vi "CRYWindow WAIT FRAME.vi"(7 "sAction":string, 10 "vi reference":refnum<vi>) -> (1 "sData_Out":string)   [LabVIEW 2013]
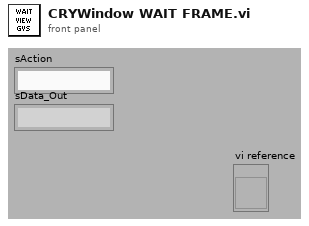
[diagram p1: front panel]
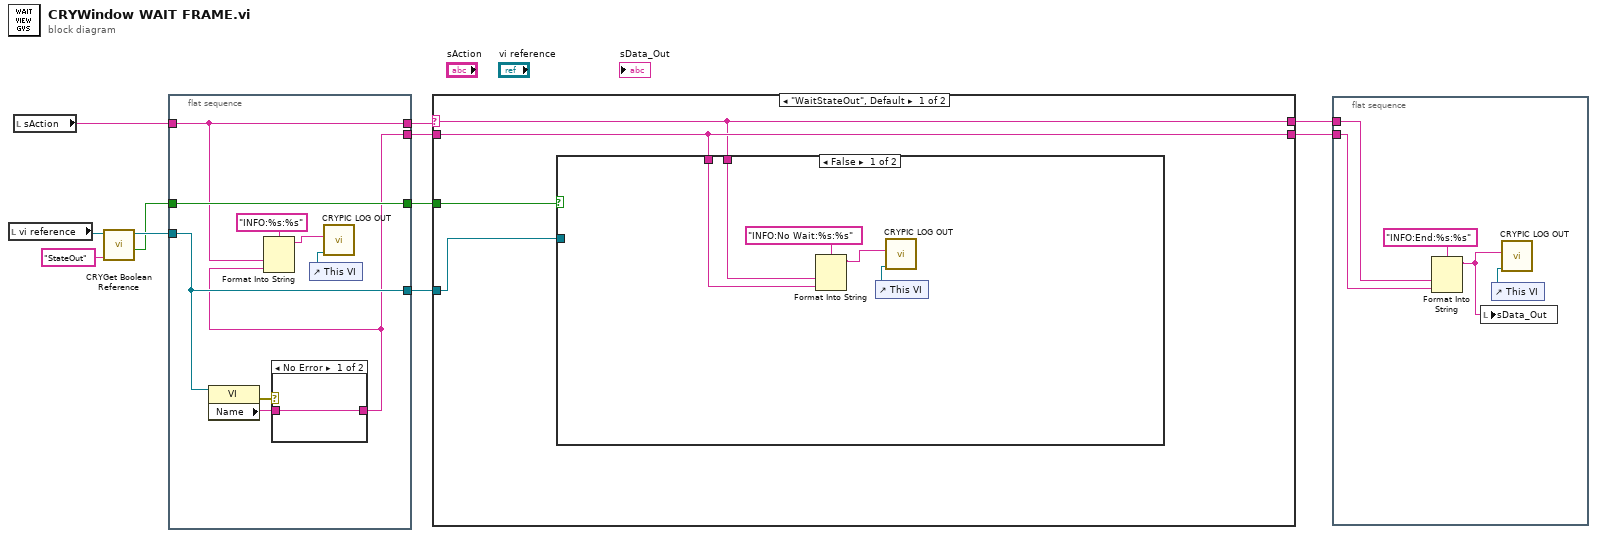
[diagram p0: block diagram]
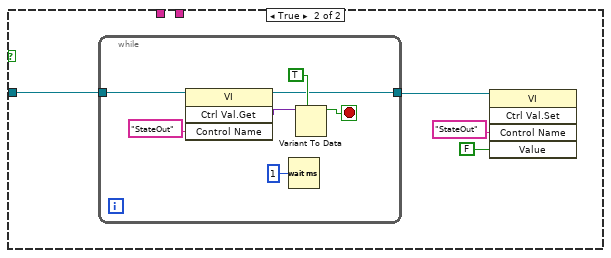
[diagram p2: hidden frame]
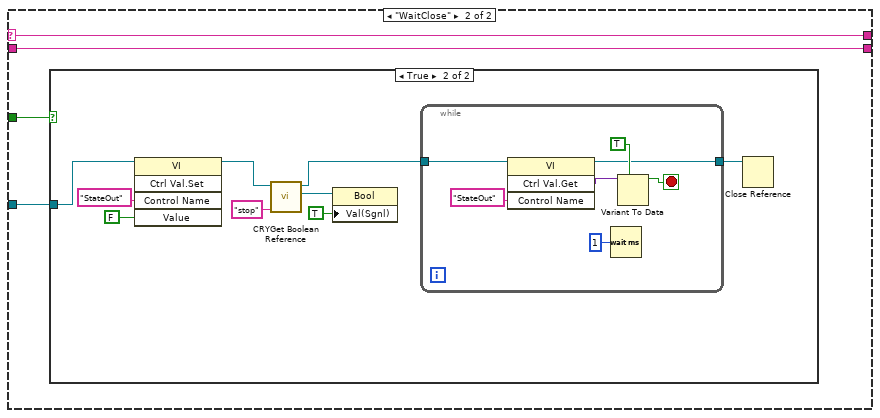
[diagram p3: hidden frame]
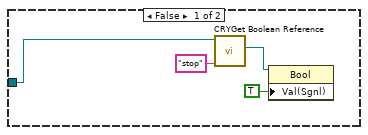
[diagram p4: hidden frame]
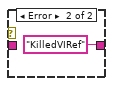
[diagram p5: hidden frame]
diagram:
  n1 = local read "vi reference"() -> (w6:refnum<vi>)
  n2 = local read "sAction"() -> (w5:string)
  n3 = call "CRYGet Boolean Reference.vi"("Label Name"="StateOut", "VI Refnum"=w6) -> ("Exist?"=w9:bool, "VI Refnum Out"=w10:refnum<vi>)  [unwired: 7 in, 1 out]
  n4 = flat-sequence {
    tunnel: [w16] -> w8
    tunnel: w10 -> [w16]
    tunnel: [w20] -> w7
    tunnel: w9 -> [w20]
    tunnel: w5 -> [w15]
    tunnel: [w15] -> w4
    tunnel: [w14] -> w2
    frame #0 {
      n5 = property class="VI"(reference=w16) -> (error out=w18:errorcluster, "Name"=w17:string)  [unwired: 1 in, 1 out]
      n6 = case shown="No Error" w18 {
        tunnel: w17 -> [w21 _]
        tunnel: [w21 "KilledVIRef" ("sAction")] -> w14
        frame No Error {
        }
        frame Error {
        }
      }
      n7 = Format Into String(format string="INFO:%s:%s" ("string"), w15, w14) -> (resulting string=w13:string)  [unwired: 2 in, 1 out]
      n8 = control-ref of="This VI"() -> (w12:refnum<vi>)
      n9 = call "CRYPIC LOG OUT.vi"("pVIRef"=w12, "sData"=w13) -> ()  [unwired: 10 in]
    }
  }
  n10 = case shown="\"WaitStateOut\", Default" w4 {
    selector: w4 -> [w23 w44]
    tunnel: w8 -> [w26 w46]
    tunnel: w7 -> [w25 w45]
    tunnel: [w23 w44] -> w3
    tunnel: w2 -> [w24 w43]
    tunnel: [w24 w43] -> w1
    frame "WaitStateOut", Default {
      n11 = case shown="False" w25 {
        tunnel: w26 -> [_ w35]
        tunnel: w24 -> [w28 _]
        tunnel: w23 -> [w27 _]
        frame False {
          n12 = Format Into String(format string="INFO:No Wait:%s:%s" ("string"), w27, w28) -> (resulting string=w30:string)  [unwired: 2 in, 1 out]
          n13 = control-ref of="This VI"() -> (w29:refnum<vi>)
          n14 = call "CRYPIC LOG OUT.vi"("pVIRef"=w29, "sData"=w30) -> ()  [unwired: 10 in]
        }
        frame True {
          n15 = while {
            tunnel: w35 -> [w41]
            tunnel: [w36] -> w32
            stop <- w38 stop-if-true
            n16 = invoke class="VI" method="Ctrl Val.Get"(reference=w41, "Control Name"="StateOut") -> (reference out=w36:refnum<vi>, "Get Control Value Variant"=w40:variant)  [unwired: 2 in, 2 out]
            n17 = Wait (ms)(milliseconds to wait=u32 1) -> ()  [unwired: 1 out]
            n18 = Variant To Data(type=TRUE, Variant=w40) -> (data=w38:bool)  [unwired: 1 in, 1 out]
          }
          n19 = invoke class="VI" method="Ctrl Val.Set"(reference=w32, "Control Name"="StateOut", "Value"=FALSE) -> ()  [unwired: 2 in, 5 out]
        }
      }
    }
    frame "WaitClose" {
      n20 = case shown="True" w45 {
        tunnel: w46 -> [w47 w52]
        frame False {
          n21 = call "CRYGet Boolean Reference.vi"("Label Name"="stop", "VI Refnum"=w47) -> ("Boolean Ref"=w50:refnum<vi>)  [unwired: 7 in, 2 out]
          n22 = property class="Bool"(reference=w50, "Val(Sgnl)"=TRUE) -> ()  [unwired: 1 in, 2 out]
        }
        frame True {
          n23 = invoke class="VI" method="Ctrl Val.Set"(reference=w52, "Control Name"="StateOut", "Value"=FALSE) -> (reference out=w54:refnum<vi>)  [unwired: 2 in, 4 out]
          n24 = call "CRYGet Boolean Reference.vi"("Label Name"="stop", "VI Refnum"=w54) -> ("Boolean Ref"=w57:refnum<vi>, "VI Refnum Out"=w53:refnum<vi>)  [unwired: 7 in, 1 out]
          n25 = property class="Bool"(reference=w57, "Val(Sgnl)"=TRUE) -> ()  [unwired: 1 in, 2 out]
          n26 = while {
            tunnel: w53 -> [w65]
            tunnel: [w60] -> w51
            stop <- w62 stop-if-true
            n27 = invoke class="VI" method="Ctrl Val.Get"(reference=w65, "Control Name"="StateOut") -> (reference out=w60:refnum<vi>, "Get Control Value Variant"=w64:variant)  [unwired: 2 in, 2 out]
            n28 = Wait (ms)(milliseconds to wait=u32 1) -> ()  [unwired: 1 out]
            n29 = Variant To Data(type=TRUE, Variant=w64) -> (data=w62:bool)  [unwired: 1 in, 1 out]
          }
          n30 = Close Reference(reference=w51) -> ()  [unwired: 1 in, 1 out]
        }
      }
    }
  }
  n31 = flat-sequence {
    tunnel: w3 -> [w70]
    tunnel: w1 -> [w69]
    frame #0 {
      n32 = Format Into String(format string="INFO:End:%s:%s" ("string"), w70, w69) -> (resulting string=w68:string)  [unwired: 2 in, 1 out]
      n33 = local write "sData_Out"(w68) -> ()
      n34 = control-ref of="This VI"() -> (w67:refnum<vi>)
      n35 = call "CRYPIC LOG OUT.vi"("pVIRef"=w67, "sData"=w68) -> ()  [unwired: 10 in]
    }
  }
